vi "Write Configuration.vi"(8 "error in (no error)":errorcluster, 10 "Configuration.lvlibp:Configuration.lvclass":refnum<class "Configuration.lvclass">, 11 "H-Intfc in":refnum<class "REST Interface.lvclass">) -> (0 "error out":errorcluster, 3 "H-Intfc out":refnum<class "REST Interface.lvclass">)   [LabVIEW 2018, in "REST Interface.lvlib" / "REST Interface.lvclass"]
uses:
  REST Interface.lvclass
  PPLs/Configuration/Configuration.lvlibp/Configuration.lvclass
  REST Interface.lvclass/REST Interface.ctl
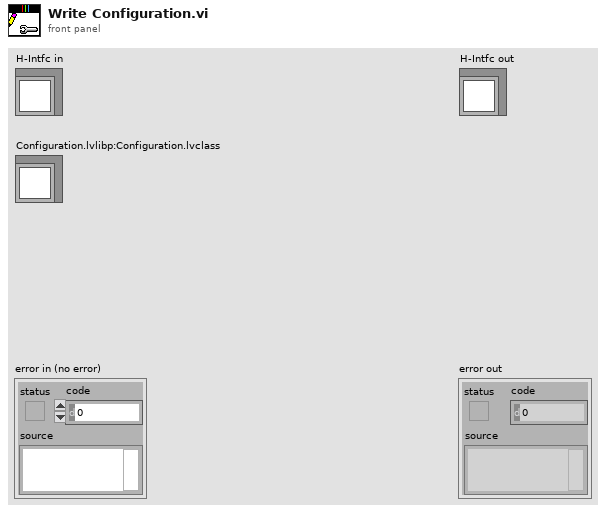
[diagram p1: front panel]
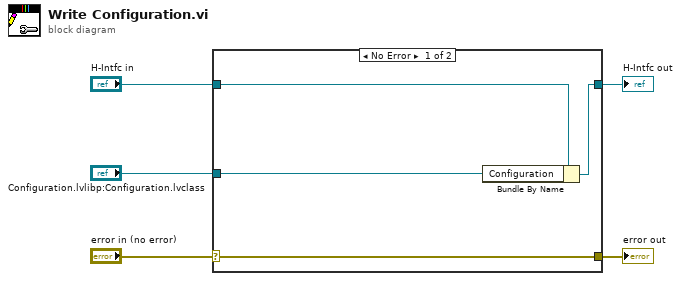
[diagram p0: block diagram]
diagram:
  n1 = case shown="No Error" "error in (no error)" {
    selector: "error in (no error)" -> [w9 w10]
    tunnel: [w9 w10] -> w4
    tunnel: [w7 w11] -> w2
    tunnel: "H-Intfc in" -> [w8 w11]
    tunnel: "Configuration.lvlibp:Configuration.lvclass" -> [w6 _]
    frame No Error {
      n2 = Bundle By Name(cluster=w8, "Configuration"=w6) -> (w7:refnum<class "REST Interface.lvclass">)
    }
    frame Error {
    }
  }
  "error out" <- w4
  "H-Intfc out" <- w2
